vi "Command Turn to Heading.vi"(2 "All Robot Commands In":T1, 3 "Startup":bool, 4 "Cmd Parameter 4":string, 5 "Cmd Parameter 3":dbl, 6 "Cmd Parameter 2":dbl, 7 "Cmd Parameter 1":dbl) -> (0 "All Robot Commands Out":T1, 1 "Completed":bool)   [LabVIEW 2016]
uses:
  Subsystems/All Robot Commands.ctl
  Subsystems/Drive and Climb SS/Drive + Climb Commands 2017.ctl
  Subsystems/Gear Delivery SS/Gear Delivery Commands.ctl
  Subsystems/Conveyor and Shooter SS/Conveyor and Shooter Commands.ctl
  Subsystems/Ball Intake SS/Ball Intake Commands.ctl
  Command Execution State.ctl
  <vilib>/Rock Robotics/WPI/ThirdParty/Sensors/Pigeon IMU/CTRE_PigeonIMU_TareType.ctl
  Global Variables/Robot Status.vi
  Global Variables/Refnum Names.vi
  Global Variables/Turn to Heading Calibrations.vi
  Global Variables/Sensor Data.vi
panel:
  out "Right F":dbl
  out "Right D":dbl
  out "Right I":dbl
  out "Right P":dbl
  out "Left F":dbl
  out "Left D":dbl
  out "Left I":dbl
  out "Left P":dbl
  out "Robot Heading":dbl
  out "Velocities":T6(graph)
  out "PID Tracking":T7(graph)
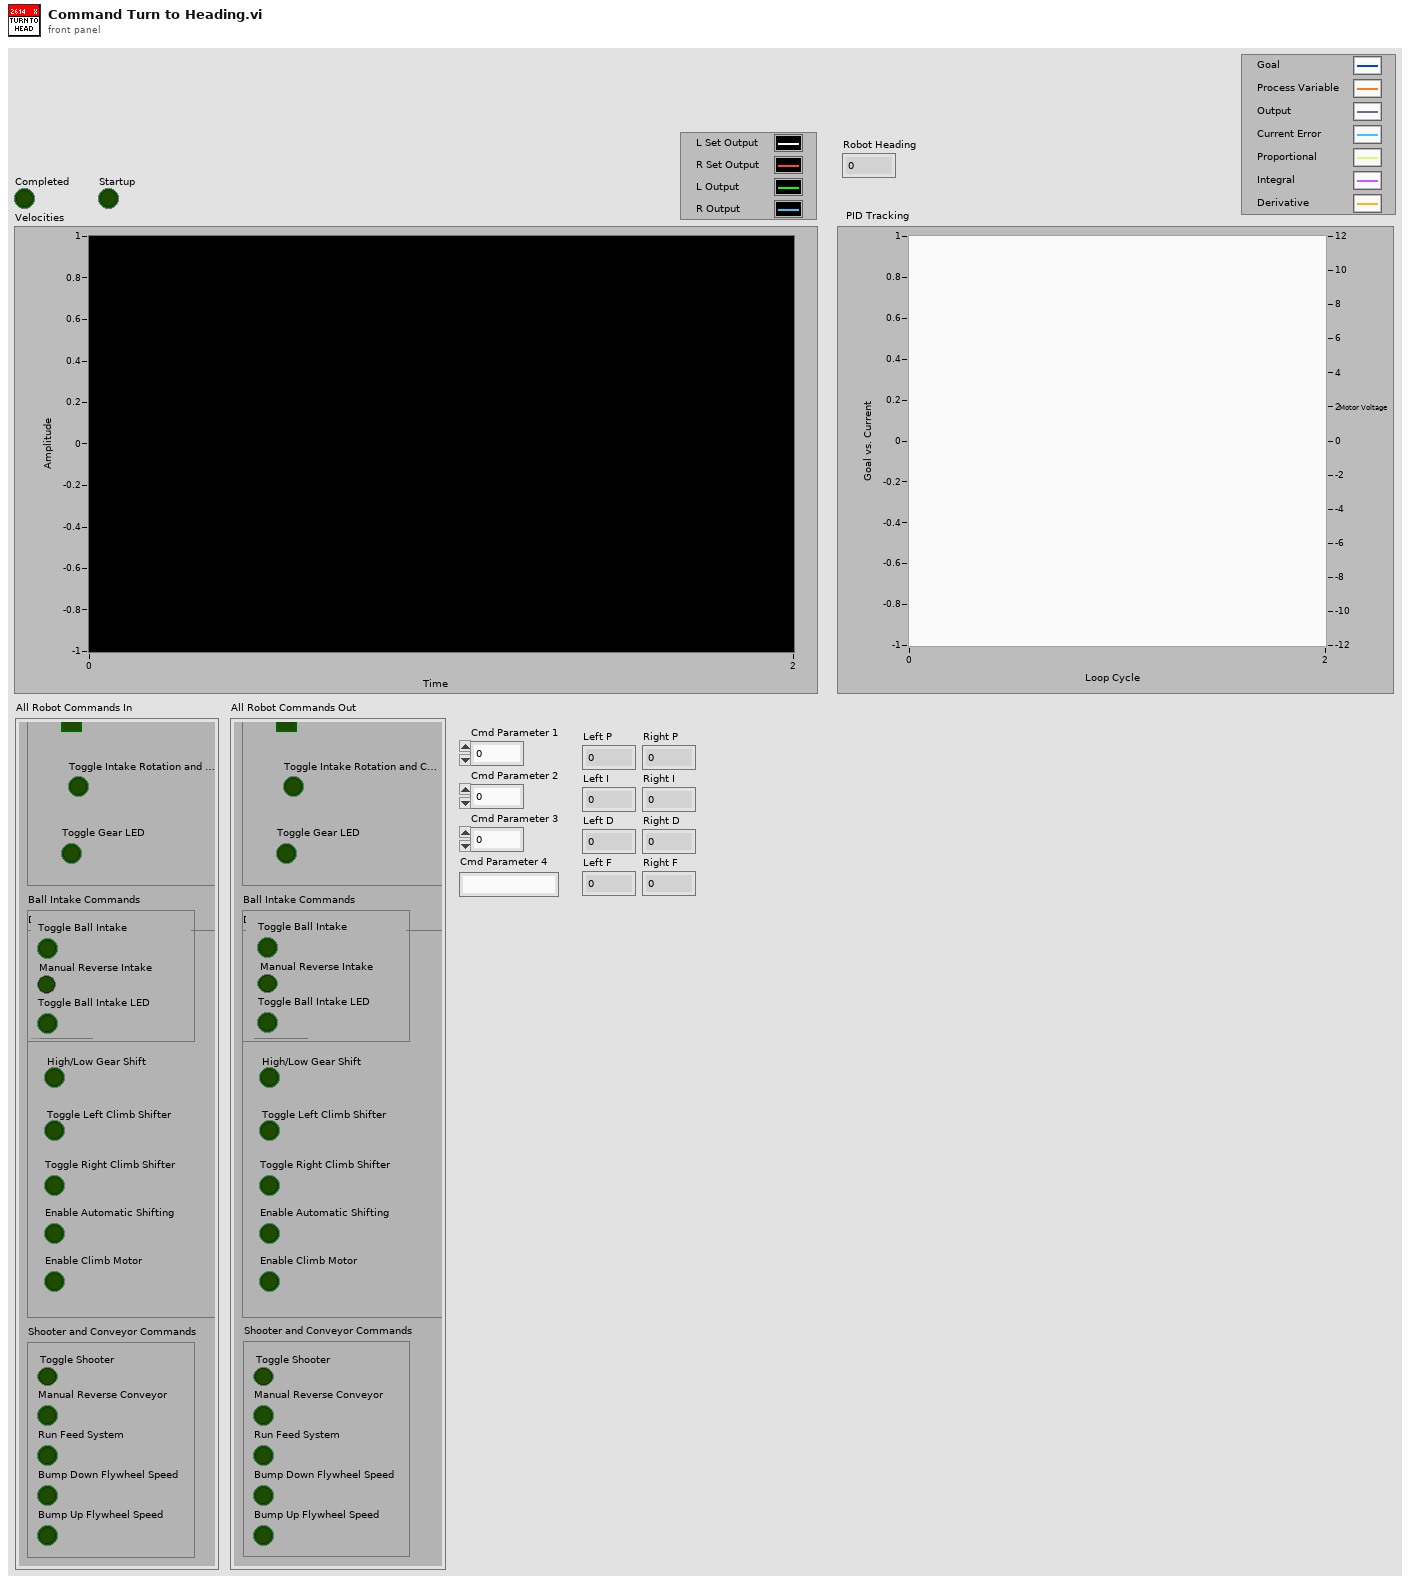
[diagram p1: front panel]
types:
  T1 = typedef "All Robot Commands.ctl" = cluster{"Drive/Climb Commands":T2, "Gear Delivery Commands":T3, "Shooter and Conveyor Commands":T4, "Ball Intake Commands":T5}
  T2 = typedef "Drive + Climb Commands 2017.ctl" = cluster{"Robot Forward-Back":dbl, "Robot Twist":dbl, "High/Low Gear Shift":bool, "Toggle Left Climb Shifter":bool, "Toggle Right Climb Shifter":bool, "Enable Automatic Shifting":bool, "Enable Climb Motor ":bool}
  T3 = typedef "Gear Delivery Commands.ctl" = cluster{"Toggle Gear Release":bool, "Toggle Intake Rotation and Chute Door":bool, "Toggle Gear LED":bool}
  T4 = typedef "Conveyor and Shooter Commands.ctl" = cluster{"Toggle Shooter":bool, "Manual Reverse Conveyor":bool, "Run Feed System":bool, "Bump Down Flywheel Speed":bool, "Bump Up Flywheel Speed":bool}
  T5 = typedef "Ball Intake Commands.ctl" = cluster{"Toggle Ball Intake":bool, "Manual Reverse Intake":bool, "Toggle Ball Intake LED":bool}
  T6 = cluster{"Left Motor Value":dbl, "Right Motor Value":dbl, "Sensor Velocity":dbl, "Sensor Velocity":dbl}
  T7 = cluster{"Goal":dbl, "Process Variable":dbl, "Max Ouput":dbl, dbl, dbl, dbl, dbl}
  T8 = typedef "Command Execution State.ctl" = enum16{"Initialize", "Execute", "Finish"}
  T9 = typedef "CTRE_PigeonIMU_TareType.ctl" = u8
  T10 = typedef "CTRE_PigeonIMU_DeviceRef.ctl" = cluster{"DeviceStatus":errorcluster, "Device Number":u8, "Type":T11, "Device ID":u32}
  T11 = typedef "CTRE_PigeonIMU_ConnectionType.ctl" = u32
  T12 = typedef "WPI_MotorControlDeviceRef.ctl" = cluster{"DeviceStatus":errorcluster, "Type":T13, "PWM":cluster{"PWM Channel":T14, "DeadBand":T15}, "CAN":cluster{"Device Number":u8, "SetOutput VI Ref":variant, "GetOutput VI Ref":variant, "Enable VI Ref":variant, "Disable VI Ref":variant, "Data":variant}, "Invert":bool}
  T13 = typedef "WPI_MotorControlType.ctl" = enum16{"PWM", "CAN"}
  T14 = typedef "FPGA_DIOPWMChannel.ctl" = enum8{"PWM 0", "PWM 1", "PWM 2", "PWM 3", "PWM 4", "PWM 5", "PWM 6", "PWM 7", "PWM 8", "PWM 9", "PWM MXP 0", "PWM MXP 1", "PWM MXP 2", "PWM MXP 3", "PWM MXP 4", "PWM MXP 5", "PWM MXP 6", "PWM MXP 7", "PWM MXP 8", "PWM MXP 9", "Invalid"}
  T15 = typedef "WPI_PWMDeadband.ctl" = cluster{"Name":string, "maxPositivePwm":i32, "minPositivePwm":i32, "centerPwm":i32, "maxNegativePwm":i32, "minNegativePwm":i32, "angularRange":u16}
  T16 = typedef "WPI_CANTalonSRX_GlobalStatus.ctl" = cluster{"Applied Throttle":dbl, "Module Enabled":bool, "CAN Error":errorcluster, "Closed Loop Error":dbl, "Forward Limit Switch Closed":bool, "Reverse Limit Switch Closed":bool, "Sensor Position":dbl, "Sensor Velocity":dbl, "Current":dbl, "Sticky Fault - Over Temp":bool, "Sticky Fault - Under Voltage":bool, "Sticky Fault - Forward Limit":bool, "Sticky Fault - Reverse Limit":bool, "Sticky Fault - Forward Soft Limit":bool, "Sticky Fault - Reverse Soft Limit":bool, "Brake is Enabled":bool, "Encoder Position":dbl, "Encoder Velocity":dbl, "Encoder Index Count":dbl, "Encoder A Pin State":bool, "Encoder B Pin State":bool, "Encoder Index Pin State":bool, "Analog In":dbl, "Analog In Velocity":dbl, "Temperature (C)":dbl, "Battery Voltage":dbl, "Control 5 Is Supported":bool, "Current Profile Slot Select":dbl, "Pos Div 8":bool, "Vel Div 4":bool, "Pulse Width Position":i32, "Pulse Width Velocity":i32, "Pulse Width Rise To Rise (us)":i32, "Pulse Width Rise To Fall (us)":i32, "Mot Prof Active Is Under Run":bool, "Mot Prof Active Has Under Run":bool, "Mot Prof Active Is Last":bool, "Mot Prof Active Velocity Only":bool, "Mot Prof Active Is Valid":bool, "Mot Prof Buffer Is Full":bool, "Mot Prof Active Profile Slot Select":i32, "Mot Prof NextID":i32, "Mot Prof Count":i32, "Mot Prof Active Velocity":dbl, "Mot Prof Active Position":dbl, "Mot Prof Output Enable":i32, "UsageFrame":u32, "Motion Magic Active Trajectory":cluster{"Velocity":dbl, "Position":dbl}}
  T17 = cluster{"Left Motor Value":dbl, "Right Motor Value":dbl, dbl, "Sensor Velocity":dbl}
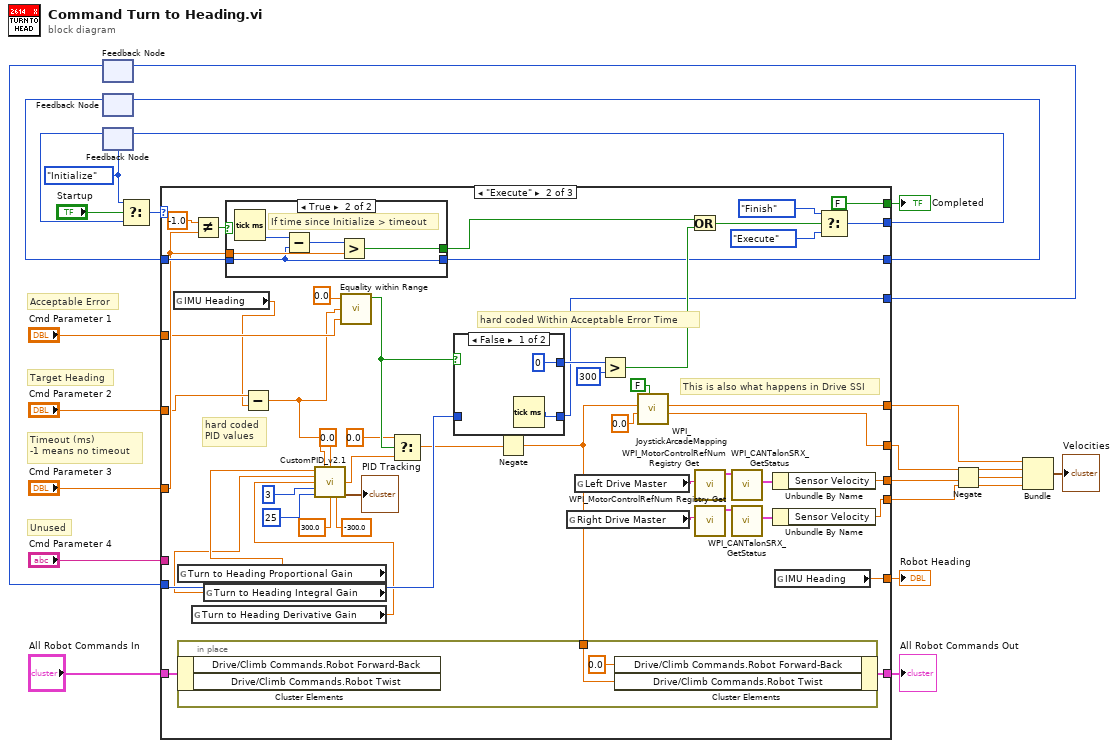
[diagram p0: block diagram]
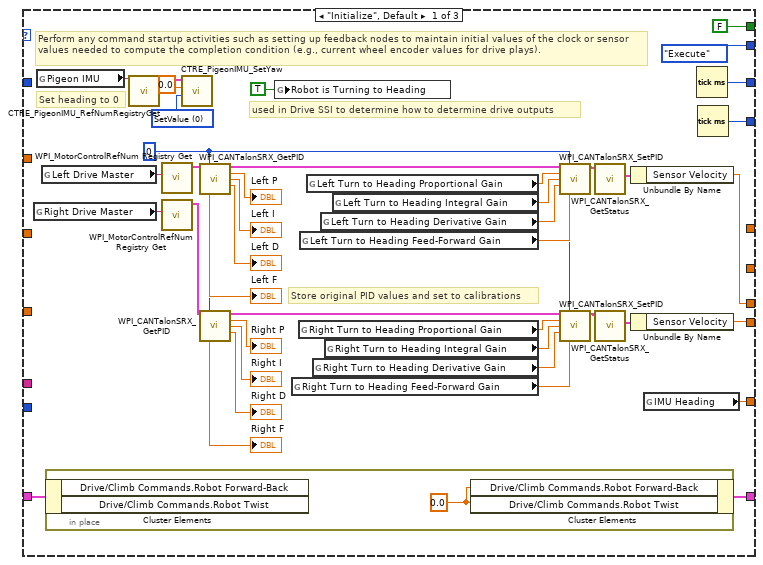
[diagram p2: hidden frame]
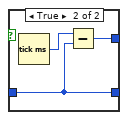
[diagram p4: hidden frame]
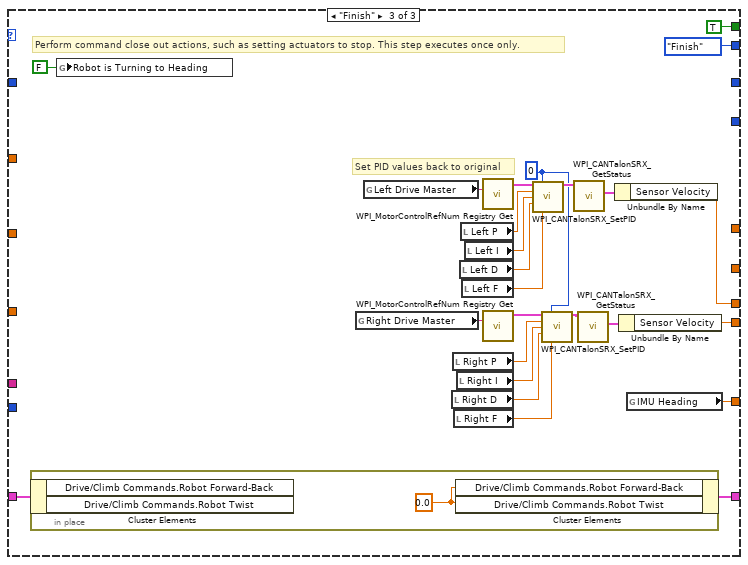
[diagram p5: hidden frame]
diagram:
  w9 = Command_Execution_State."Initialize" ("Play State")
  # "Unused"
  # "Timeout (ms)\n-1 means no timeout"
  # "Target Heading"
  # "Acceptable Error"
  n1 = feedback #1() -> (w14:u32)  [unwired: 1 in]
  n2 = feedback #2() -> (w16:u32)  [unwired: 1 in]
  n3 = feedback #3(w9) -> (w11:T8)
  n4 = Select(t=w9, s="Startup", f=w11) -> (s? t:f=w10:T8)
  n5 = case shown="\"Execute\"" w10 {
    tunnel: [FALSE FALSE TRUE] -> w23
    tunnel: [Command_Execution_State."Execute" ("Play State") w114 Command_Execution_State."Finish" ("f")] -> w22
    tunnel: "Cmd Parameter 1" -> [_ w96 _]
    tunnel: "Cmd Parameter 2" -> [_ w72 _]
    tunnel: "Cmd Parameter 3" -> [_ w99 _]
    tunnel: "Cmd Parameter 4" -> [_ _ _]
    tunnel: w16 -> [_ w106 _]
    tunnel: [w62 w97 _] -> w17
    tunnel: [w61 w101 _] -> w15
    tunnel: w14 -> [_ w76 _]
    tunnel: [w30 w88 w136] -> w13
    tunnel: [w58 w78 w135] -> w12
    tunnel: [w32 w77 w130] -> w7
    tunnel: [w33 w86 w133] -> w6
    tunnel: "All Robot Commands In" -> [w34 w87 w134]
    tunnel: [_ w80 _] -> w4
    tunnel: [_ w79 _] -> w3
    frame "Initialize", Default {
      w27 = T9 0 items=["SetValue"=0, "AddOffset"=1, "MatchCompass"=2, "SetOffset"=255] ("TareType (SetValue)")
      w31 = u8 0 ("Parameter Slot")
      # "Store original PID values and set to calibrations"
      # "used in Drive SSI to determine how to determine drive outputs"
      # "Set heading to 0"
      # "Perform any command startup activities such as setting up feedback nodes to maintain initial values of the clock or sensor values needed to compute the completion condition (e.g., current wheel encoder values for drive plays)."
      n6 = global read "Refnum Names.vi" "Right Drive Master"() -> (w57:string)
      n7 = global read "Refnum Names.vi" "Pigeon IMU"() -> (w26:string)
      n8 = global read "Refnum Names.vi" "Left Drive Master"() -> (w56:string)
      n9 = in-place {
        w65 = 0.0 ("Drive/Climb Commands.Robot Twist")
        n10 = in-place-cluster #4(w34) -> ()  [unwired: 2 out]
        n11 = in-place-cluster #4("Drive/Climb Commands.Robot Forward-Back"=w65, "Drive/Climb Commands.Robot Twist"=w65) -> (w33:T1)
      }
      n12 = call <vilib>:"CTRE_PigeonIMU_RefNumRegistryGet.vi"("refnum name"=w26) -> ("PigeonIMUDevRef"=w25:T10)  [unwired: 9 in, 1 out]
      n13 = call <vilib>:"WPI_MotorControlRefNum Registry Get.vi"("refnum name"=w56) -> ("MotorControlDevRef"=w47:T12)  [unwired: 9 in, 1 out]
      n14 = call <vilib>:"WPI_MotorControlRefNum Registry Get.vi"("refnum name"=w57) -> ("MotorControlDevRef"=w37:T12)  [unwired: 9 in, 1 out]
      n15 = call <vilib>:"CTRE_PigeonIMU_SetYaw.vi"("TareType (SetValue)"=w27, "Value"=0.0, "PigeonIMUDevRef"=w25) -> ()  [unwired: 7 in, 2 out]
      n16 = call <vilib>:"WPI_CANTalonSRX_GetPID.vi"("CAN Talon SRX Ref"=w47, "Parameter Slot"=w31) -> ("CAN Talon SRX Ref"=w54:T12, "P"=→"Left P":dbl, "I"=→"Left I":dbl, "D"=→"Left D":dbl, "F"=→"Left F":dbl)  [unwired: 6 in, 3 out]
      n17 = call <vilib>:"WPI_CANTalonSRX_GetPID.vi"("CAN Talon SRX Ref"=w37, "Parameter Slot"=w31) -> ("CAN Talon SRX Ref"=w36:T12, "P"=→"Right P":dbl, "I"=→"Right I":dbl, "D"=→"Right D":dbl, "F"=→"Right F":dbl)  [unwired: 6 in, 3 out]
      n18 = global write "Robot Status.vi" "Robot is Turning to Heading"(TRUE ("Robot is Turning to Heading")) -> ()
      n19 = global read "Turn to Heading Calibrations.vi" "Right Turn to Heading Feed-Forward Gain"() -> (w38:dbl)
      n20 = global read "Turn to Heading Calibrations.vi" "Right Turn to Heading Proportional Gain"() -> (w41:dbl)
      n21 = global read "Turn to Heading Calibrations.vi" "Left Turn to Heading Feed-Forward Gain"() -> (w48:dbl)
      n22 = global read "Turn to Heading Calibrations.vi" "Left Turn to Heading Proportional Gain"() -> (w51:dbl)
      n23 = global read "Turn to Heading Calibrations.vi" "Right Turn to Heading Derivative Gain"() -> (w39:dbl)
      n24 = global read "Turn to Heading Calibrations.vi" "Left Turn to Heading Derivative Gain"() -> (w49:dbl)
      n25 = global read "Turn to Heading Calibrations.vi" "Right Turn to Heading Integral Gain"() -> (w40:dbl)
      n26 = global read "Turn to Heading Calibrations.vi" "Left Turn to Heading Integral Gain"() -> (w50:dbl)
      n27 = call <vilib>:"WPI_CANTalonSRX_SetPID.vi"("CAN Talon SRX Ref"=w54, "Parameter Slot"=w31, "P"=w51, "I"=w50, "D"=w49, "F"=w48) -> ("CAN Talon SRX Ref"=w46:T12)  [unwired: 8 in, 1 out]
      n28 = call <vilib>:"WPI_CANTalonSRX_SetPID.vi"("CAN Talon SRX Ref"=w36, "Parameter Slot"=w31, "P"=w41, "I"=w40, "D"=w39, "F"=w38) -> ("CAN Talon SRX Ref"=w35:T12)  [unwired: 8 in, 1 out]
      n29 = call <vilib>:"WPI_CANTalonSRX_GetStatus.vi"("CAN Talon SRX Ref"=w46) -> ("Talon SRX Status"=w60:T16)  [unwired: 8 in, 2 out]
      n30 = call <vilib>:"WPI_CANTalonSRX_GetStatus.vi"("CAN Talon SRX Ref"=w35) -> ("Talon SRX Status"=w59:T16)  [unwired: 8 in, 2 out]
      n31 = Unbundle By Name(w60) -> ("Sensor Velocity"=w30:dbl)
      n32 = Unbundle By Name(w59) -> ("Sensor Velocity"=w58:dbl)
      n33 = global read "Sensor Data.vi" "IMU Heading"() -> (w32:dbl)
      n34 = Tick Count (ms)() -> (millisecond timer value=w62:u32)
      n35 = Tick Count (ms)() -> (millisecond timer value=w61:u32)
    }
    frame "Execute" {
      # "This is also what happens in Drive SSI"
      # "hard coded\nPID values"
      # "hard coded Within Acceptable Error Time"
      n36 = global read "Sensor Data.vi" "IMU Heading"() -> (w71:dbl)
      n37 = global read "Turn to Heading Calibrations.vi" "Turn to Heading Proportional Gain"() -> (w68:dbl)
      n38 = global read "Turn to Heading Calibrations.vi" "Turn to Heading Derivative Gain"() -> (w66:dbl)
      n39 = Not Equal?(x=-1.0 ("y"), y=w99) -> (x != y?=w107:bool)
      n40 = global read "Turn to Heading Calibrations.vi" "Turn to Heading Integral Gain"() -> (w67:dbl)
      n41 = case shown="True" w107 {
        selector: w107 -> [w119 _]
        tunnel: [w119 w123] -> w83
        tunnel: w106 -> [w118 w120]
        tunnel: w99 -> [_ w122]
        tunnel: [w118 w120] -> w97
        frame False {
          # "If param 3 is -1, this is always false"
        }
        frame True {
          # "If time since Initialize > timeout"
          n42 = Tick Count (ms)() -> (millisecond timer value=w124:u32)
          n43 = Subtract(x=w124, y=w120) -> (x-y=w121:u32)
          n44 = Greater?(x=w121, y=w122) -> (0:w123:bool)
        }
      }
      n45 = Subtract(x=w72, y=w71) -> (x-y=w70:dbl)
      n46 = call "CustomPID_v2.1.vi"("Kp"=w68, "Process Variable"=w70, "Goal"=0.0, "Ki"=w67, "Kd"=w66, "N-Diff"=3, "N-Int"=25, "Max Ouput"=300.0, "Min Output"=-300.0) -> ("Command"=w90:dbl, "PID Tracking"=→"PID Tracking":T7)  [unwired: 4 in, 1 out]
      n47 = call "Equality within Range.vi"("Range"=w96, "Y"=w70, "X"=0.0) -> ("X = Y within Range?"=w105:bool)
      n48 = Select(t=0.0, s=w105, f=w90) -> (s? t:f=w75:dbl)
      n49 = case shown="False" w105 {
        tunnel: [w125 w127] -> w101
        tunnel: [0 w129] -> w102
        tunnel: w76 -> [_ w127]
        frame False {
          n50 = Tick Count (ms)() -> (millisecond timer value=w125:u32)
        }
        frame True {
          n51 = Tick Count (ms)() -> (millisecond timer value=w128:u32)
          n52 = Subtract(x=w128, y=w127) -> (x-y=w129:u32)
        }
      }
      n53 = Negate(x=w75) -> (-x=w69:dbl)
      n54 = in-place {
        in-place-border: w69 -> [w117]
        n55 = in-place-cluster #5(w87) -> ()  [unwired: 2 out]
        n56 = in-place-cluster #5("Drive/Climb Commands.Robot Forward-Back"=0.0, "Drive/Climb Commands.Robot Twist"=w117) -> (w86:T1)
      }
      n57 = global read "Refnum Names.vi" "Right Drive Master"() -> (w84:string)
      n58 = global read "Refnum Names.vi" "Left Drive Master"() -> (w85:string)
      n59 = Greater?(x=w102, y=u32 300) -> (0:w103:bool)
      n60 = call <vilib>:"WPI_JoystickArcadeMapping.vi"("Square Inputs"=FALSE, "Y axis value"=0.0, "X axis value"=w69) -> ("Right Motor Value"=w79:dbl, "Left Motor Value"=w80:dbl)  [unwired: 7 in]
      n61 = Or(x=w83, y=w103) -> (x .or. y?=w104:bool)
      n62 = call <vilib>:"WPI_MotorControlRefNum Registry Get.vi"("refnum name"=w85) -> ("MotorControlDevRef"=w108:T12)  [unwired: 9 in, 1 out]
      n63 = call <vilib>:"WPI_MotorControlRefNum Registry Get.vi"("refnum name"=w84) -> ("MotorControlDevRef"=w110:T12)  [unwired: 9 in, 1 out]
      n64 = call <vilib>:"WPI_CANTalonSRX_GetStatus.vi"("CAN Talon SRX Ref"=w108) -> ("Talon SRX Status"=w109:T16)  [unwired: 8 in, 2 out]
      n65 = call <vilib>:"WPI_CANTalonSRX_GetStatus.vi"("CAN Talon SRX Ref"=w110) -> ("Talon SRX Status"=w111:T16)  [unwired: 8 in, 2 out]
      n66 = Unbundle By Name(w109) -> ("Sensor Velocity"=w88:dbl)
      n67 = Unbundle By Name(w111) -> ("Sensor Velocity"=w78:dbl)
      n68 = global read "Sensor Data.vi" "IMU Heading"() -> (w77:dbl)
      n69 = Select(t=Command_Execution_State."Finish" ("Play State"), s=w104, f=Command_Execution_State."Execute" ("Play State")) -> (s? t:f=w114:T8)
    }
    frame "Finish" {
      w131 = u8 0 ("Parameter Slot")
      # "Set PID values back to original"
      # "Perform command close out actions, such as setting actuators to stop. This step executes once only."
      n70 = in-place {
        w155 = 0.0 ("Drive/Climb Commands.Robot Twist")
        n71 = in-place-cluster #6(w134) -> ()  [unwired: 2 out]
        n72 = in-place-cluster #6("Drive/Climb Commands.Robot Forward-Back"=w155, "Drive/Climb Commands.Robot Twist"=w155) -> (w133:T1)
      }
      n73 = global write "Robot Status.vi" "Robot is Turning to Heading"(FALSE ("Robot is Turning to Heading")) -> ()
      n74 = global read "Refnum Names.vi" "Right Drive Master"() -> (w150:string)
      n75 = global read "Refnum Names.vi" "Left Drive Master"() -> (w149:string)
      n76 = local read "Right D"() -> (w141:dbl)
      n77 = local read "Right P"() -> (w143:dbl)
      n78 = local read "Right F"() -> (w140:dbl)
      n79 = local read "Right I"() -> (w142:dbl)
      n80 = local read "Left D"() -> (w145:dbl)
      n81 = local read "Left P"() -> (w147:dbl)
      n82 = local read "Left F"() -> (w144:dbl)
      n83 = local read "Left I"() -> (w146:dbl)
      n84 = call <vilib>:"WPI_MotorControlRefNum Registry Get.vi"("refnum name"=w149) -> ("MotorControlDevRef"=w148:T12)  [unwired: 9 in, 1 out]
      n85 = call <vilib>:"WPI_MotorControlRefNum Registry Get.vi"("refnum name"=w150) -> ("MotorControlDevRef"=w139:T12)  [unwired: 9 in, 1 out]
      n86 = call <vilib>:"WPI_CANTalonSRX_SetPID.vi"("CAN Talon SRX Ref"=w148, "Parameter Slot"=w131, "P"=w147, "I"=w146, "D"=w145, "F"=w144) -> ("CAN Talon SRX Ref"=w137:T12)  [unwired: 8 in, 1 out]
      n87 = call <vilib>:"WPI_CANTalonSRX_SetPID.vi"("CAN Talon SRX Ref"=w139, "Parameter Slot"=w131, "P"=w143, "I"=w142, "D"=w141, "F"=w140) -> ("CAN Talon SRX Ref"=w138:T12)  [unwired: 8 in, 1 out]
      n88 = call <vilib>:"WPI_CANTalonSRX_GetStatus.vi"("CAN Talon SRX Ref"=w137) -> ("Talon SRX Status"=w151:T16)  [unwired: 8 in, 2 out]
      n89 = call <vilib>:"WPI_CANTalonSRX_GetStatus.vi"("CAN Talon SRX Ref"=w138) -> ("Talon SRX Status"=w152:T16)  [unwired: 8 in, 2 out]
      n90 = Unbundle By Name(w151) -> ("Sensor Velocity"=w136:dbl)
      n91 = Unbundle By Name(w152) -> ("Sensor Velocity"=w135:dbl)
      n92 = global read "Sensor Data.vi" "IMU Heading"() -> (w130:dbl)
    }
  }
  "Completed" <- w23
  "Robot Heading" <- w7
  "All Robot Commands Out" <- w6
  n93 = feedback-in #1(w15) -> ()
  n94 = feedback-in #2(w17) -> ()
  n95 = feedback-in #3(w22) -> ()
  n96 = Negate(x=w13) -> (-x=w1:dbl)
  n97 = Bundle("Left Motor Value"=w4, "Right Motor Value"=w3, w1, "Sensor Velocity"=w12) -> (→"Velocities":T17)  [unwired: 1 in]
